vi "NS_NoneModifing.vi"(0 "object in":refnum<class "NativeSubTemplate.lvclass">, 5 "Error In":errorcluster) -> (14 "object out":refnum<class "NativeSubTemplate.lvclass">, 19 "Error Out":errorcluster)   [LabVIEW 2020, in "NativeSubTemplate.lvclass"]
uses:
  NativeSubTemplate.lvclass
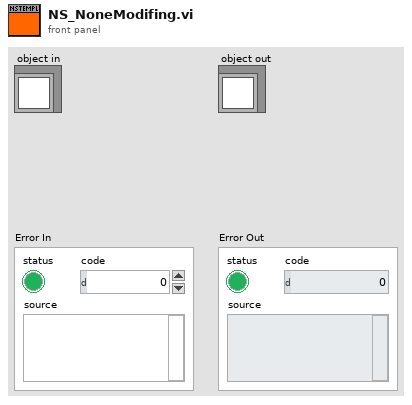
[diagram p1: front panel]
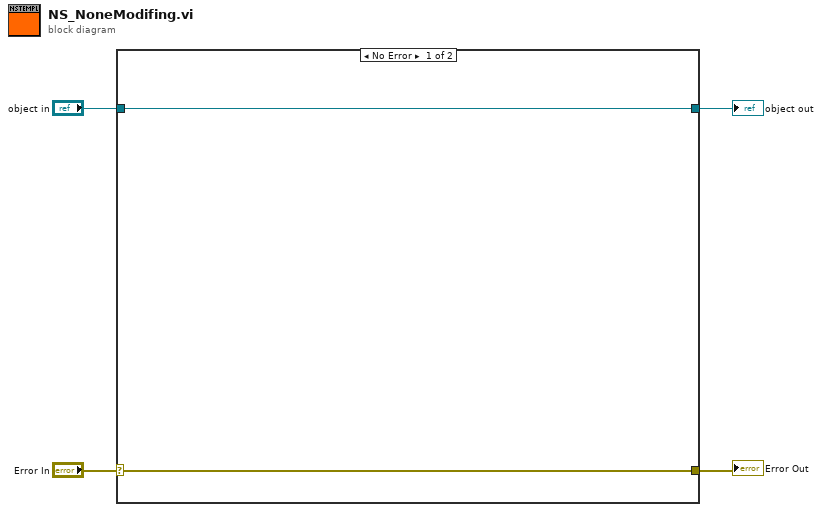
[diagram p0: block diagram]
diagram:
  n1 = case shown="No Error" "Error In" {
    selector: "Error In" -> [w5 w8]
    tunnel: [w5 w8] -> w3
    tunnel: [w6 w7] -> w1
    tunnel: "object in" -> [w6 w7]
    frame No Error {
    }
    frame Error {
    }
  }
  "Error Out" <- w3
  "object out" <- w1
